vi "Read total_income.vi"(8 "error in (no error)":errorcluster, 11 "Tax_calculation in":refnum<class "Tax_calculation.lvclass">) -> (0 "error out":errorcluster, 2 "total_income":dbl, 3 "Tax_calculation out":refnum<class "Tax_calculation.lvclass">)   [LabVIEW 2016, in "Tax_calculation.lvclass"]
uses:
  Tax_calculation.lvclass
  Tax_calculation.lvclass/Tax_calculation.ctl
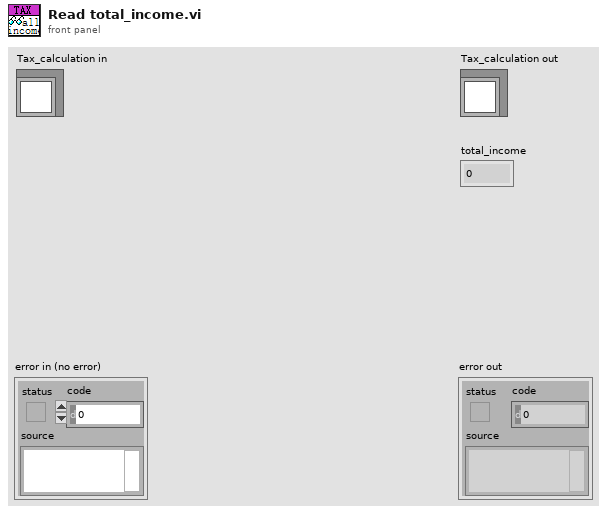
[diagram p1: front panel]
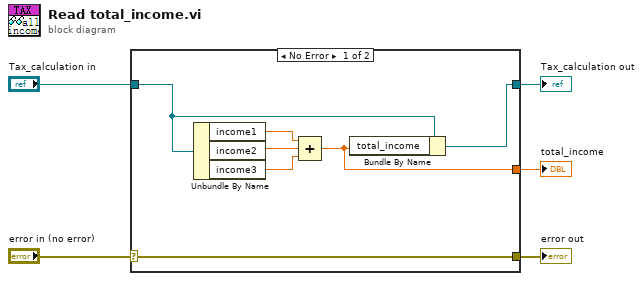
[diagram p0: block diagram]
diagram:
  n1 = case shown="No Error" "error in (no error)" {
    selector: "error in (no error)" -> [w12 w13]
    tunnel: [w12 w13] -> w4
    tunnel: [w7 w14] -> w2
    tunnel: "Tax_calculation in" -> [w8 w14]
    tunnel: [w6 _] -> w1
    frame No Error {
      n2 = Unbundle By Name(w8) -> ("income1"=w11:dbl, "income2"=w10:dbl, "income3"=w9:dbl)
      n3 = Compound Arithmetic op=ADD(w11, w10, w9) -> (w6:dbl)
      n4 = Bundle By Name(cluster=w8, "total_income"=w6) -> (w7:refnum<class "Tax_calculation.lvclass">)
    }
    frame Error {
    }
  }
  "error out" <- w4
  "Tax_calculation out" <- w2
  "total_income" <- w1
